vi "ModHeaderFileItem.vi"(8 "error in":errorcluster caption="error out", 11 "Data Path":path) -> (0 "error out":errorcluster)   [LabVIEW 2019]
uses:
  Interface Class/ScanParams.ctl
  Interface Class/ScanParamsOld.ctl
  Interface Class/Interface.lvclass
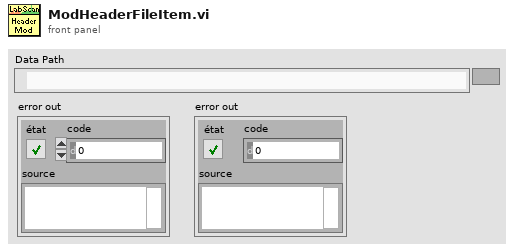
[diagram p1: front panel]
types:
  T1 = enum16{"open", "replace", "create", "open or create", "replace or create", "replace or create with confirmation"}
  T2 = typedef "Interface.lvclass/ScanParamsOld.ctl" = cluster{"Entête":string, "Scan list":string[], "NbCourbe":i32, "IndCourbe":i64, "NomDon":string[], "Session ":i32, "Date":string, "Time":string, "VarParams":string[][], "UserName":string, "ScanTableSize":i32[], "VarPar list":string[]}
  T3 = typedef "Interface.lvclass/ScanParams.ctl" = cluster{"Entête":string, "Scan list":string[], "NbCourbe":i32, "IndCourbe":i64, "NomDon":string[], "Session ":i32, "Date":string, "Time":string, "VarParams":string[][], "UserName":string, "ScanTableSize":i32[], "VarPar list":string[], "DescKeyword":string}
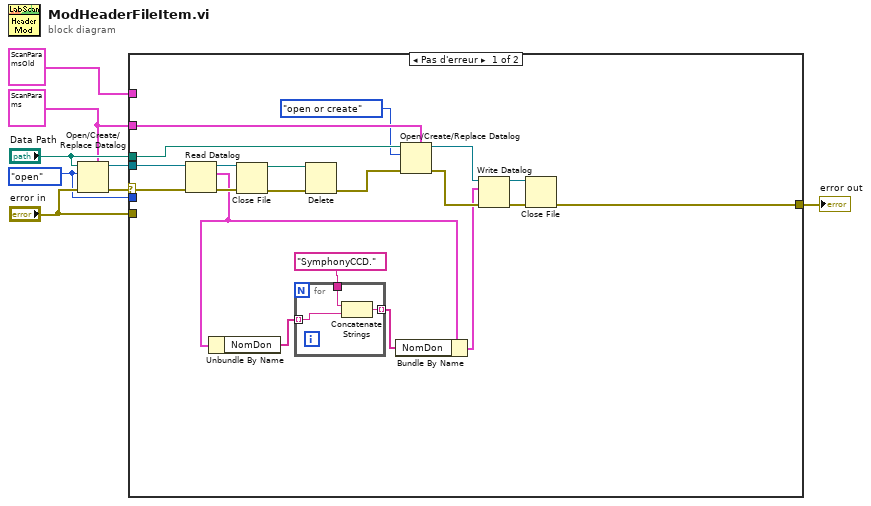
[diagram p0: block diagram]
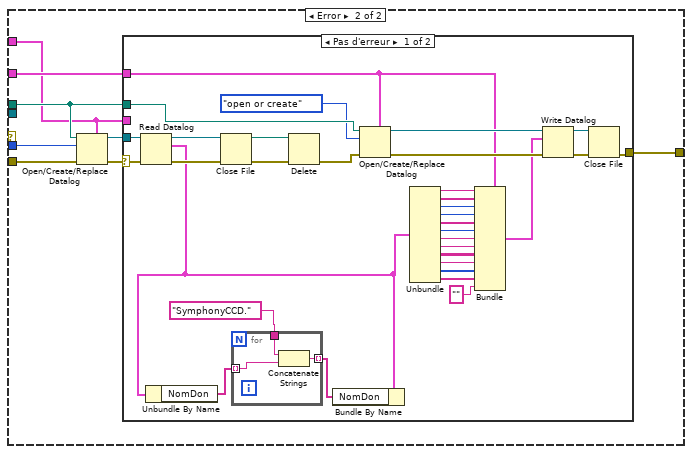
[diagram p2: hidden frame]
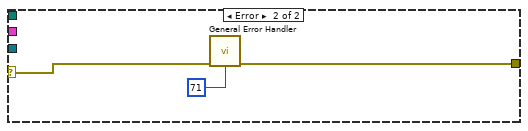
[diagram p3: hidden frame]
diagram:
  w2 = T1."open" ("opération (0 : open)")
  w6 = T3 {"Entête"="", "Scan list"=[], "NbCourbe"=1, "IndCourbe"=1, "NomDon"=["RTêta;", "X&Y;"], "Session "=0, "Date"="", "Time"="", "VarParams"=[], "UserName"="", "ScanTableSize"=[], "VarPar list"=[], "DescKeyword"=""} ("ScanParams")
  n1 = Open/Create/Replace Datalog(5:w6, 8:"error in", 10:w2, 11:"Data Path") -> (0:w4:errorcluster, 3:w3:refnum<k1>)  [unwired: 2 in, 1 out]
  n2 = case shown="Pas d'erreur" w4 {
    selector: w4 -> [w27 _]
    tunnel: "error in" -> [_ w39]
    tunnel: [w25 w36] -> w5
    tunnel: T2 {"Entête"="", "Scan list"=[], "NbCourbe"=1, "IndCourbe"=0, "NomDon"=["RTêta;", "X&Y;"], "Session "=0, "Date"="", "Time"="", "VarParams"=[], "UserName"="", "ScanTableSize"=[], "VarPar list"=[]} ("ScanParams") -> [_ w32]
    tunnel: w3 -> [w28 _]
    tunnel: "Data Path" -> [w15 w34]
    tunnel: w2 -> [_ w38]
    tunnel: w6 -> [w16 w33]
    frame No Error {
      n3 = Read Datalog(4:w27, 7:w28) -> (0:w22:errorcluster, 2:w9:T3, 3:w23:refnum<k1>)  [unwired: 1 in]
      n4 = Unbundle By Name(w9) -> ("NomDon"=w13:string[])
      n5 = Close File(refnum=w23, error in=w22) -> (path=w20:path, error out=w21:errorcluster)
      n6 = for {
        tunnel: w13 -> [w30] mode=indexing
        tunnel: "SymphonyCCD." -> [w31]
        tunnel: [w29] -> w11 mode=indexing
        n7 = Concatenate Strings(w31, w30) -> (w29:string)
      }
      n8 = Delete(path (use dialog)=w20, error in=w21) -> (error out=w19:errorcluster)  [unwired: 3 in, 2 out]
      n9 = Bundle By Name(cluster=w9, "NomDon"=w11) -> (w10:T3)
      n10 = Open/Create/Replace Datalog(5:w16, 8:w19, 10:T1."open or create" ("opération (0 : open)"), 11:w15) -> (0:w18:errorcluster, 3:w17:refnum<k1>)  [unwired: 2 in, 1 out]
      n11 = Write Datalog(4:w18, 6:w10, 7:w17) -> (0:w26:errorcluster, 3:w24:refnum<k1>)
      n12 = Close File(refnum=w24, error in=w26) -> (error out=w25:errorcluster)  [unwired: 1 out]
    }
    frame Error {
      n13 = Open/Create/Replace Datalog(5:w32, 8:w39, 10:w38, 11:w34) -> (0:w37:errorcluster, 3:w35:refnum<k1>)  [unwired: 2 in, 1 out]
      n14 = case shown="Pas d'erreur" w37 {
        selector: w37 -> [w72 w77]
        tunnel: [w69 w76] -> w36
        tunnel: w35 -> [w71 _]
        tunnel: w32 -> [_ _]
        tunnel: w34 -> [w62 _]
        tunnel: w33 -> [w54 _]
        frame No Error {
          n15 = Read Datalog(4:w72, 7:w71) -> (0:w66:errorcluster, 2:w55:T2, 3:w67:refnum<k1>)  [unwired: 1 in]
          n16 = Unbundle By Name(w55) -> ("NomDon"=w58:string[])
          n17 = Close File(refnum=w67, error in=w66) -> (path=w65:path, error out=w64:errorcluster)
          n18 = for {
            tunnel: w58 -> [w74] mode=indexing
            tunnel: "SymphonyCCD." -> [w75]
            tunnel: [w73] -> w56 mode=indexing
            n19 = Concatenate Strings(w75, w74) -> (w73:string)
          }
          n20 = Delete(path (use dialog)=w65, error in=w64) -> (error out=w61:errorcluster)  [unwired: 3 in, 2 out]
          n21 = Bundle By Name(cluster=w55, "NomDon"=w56) -> ()  [unwired: 1 out]
          n22 = Open/Create/Replace Datalog(5:w54, 8:w61, 10:T1."open or create" ("opération (0 : open)"), 11:w62) -> (0:w60:errorcluster, 3:w63:refnum<k1>)  [unwired: 2 in, 1 out]
          n23 = Unbundle(w55) -> ("Entête"=w53:string, "Scan list"=w52:string[], "NbCourbe"=w51:i32, "IndCourbe"=w50:i64, "NomDon"=w49:string[], "Session"=w48:i32, "Date"=w47:string, "Time"=w46:string, "VarParams"=w45:string[][], "UserName"=w44:string, "ScanTableSize"=w43:i32[], "VarPar list"=w42:string[])
          n24 = Bundle(cluster=w54, "Entête"=w53, "Scan list"=w52, "NbCourbe"=w51, "IndCourbe"=w50, "NomDon"=w49, "Session"=w48, "Date"=w47, "Time"=w46, "VarParams"=w45, "UserName"=w44, "ScanTableSize"=w43, "VarPar list"=w42, "DescKeyword"="") -> (w40:T3)
          n25 = Write Datalog(4:w60, 6:w40, 7:w63) -> (0:w70:errorcluster, 3:w68:refnum<k1>)
          n26 = Close File(refnum=w68, error in=w70) -> (error out=w69:errorcluster)  [unwired: 1 out]
        }
        frame Error {
          n27 = call <vilib>:"General Error Handler.vi"("error in (no error)"=w77, "[exception code]"=71) -> ("error out"=w76:errorcluster)  [unwired: 9 in, 4 out]
        }
      }
    }
  }
  "error out" <- w5
